vi "Target VI Read.vi"(4 "error in (no error)":errorcluster, 6 "Container State":T2, 7 "Display State In":T1) -> (0 "error out":errorcluster, 2 "Value":path, 3 "Display State Out":T1)   [LabVIEW 2009, in "Jump Button (Modern).xctl"]
uses:
  <vilib>/Navigation Controls/Jump Button/Jump Button (Modern).xctl
  <vilib>/_xctls/Container State.ctl
  <vilib>/Navigation Controls/Jump Button/Jump Button State.ctl
  <vilib>/Navigation Controls/NI_Navigation.lvlib
  <vilib>/_xctls/XControlSupport.lvlib
panel:
  # "Replace the Value Indicator below with an Indicator of desired type.\nDo not remove this Indicator or the others from the connector pane. \nDo not change the connector pane pattern.\nThe Value Indicator should always be the second terminal from top on the output side in the connector pane."
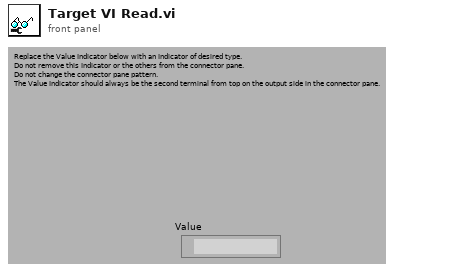
[diagram p1: front panel]
types:
  T1 = typedef "Jump Button (Modern).xctl/Jump Button State.ctl" = cluster{"Button Text":string, "Absolute Path":path, "Relative Path":path}
  T2 = typedef "XControlSupport.lvlib/Container State.ctl" = cluster{"Indicator?":bool, "Run Mode?":bool, " Refnum":refnum<vi>}
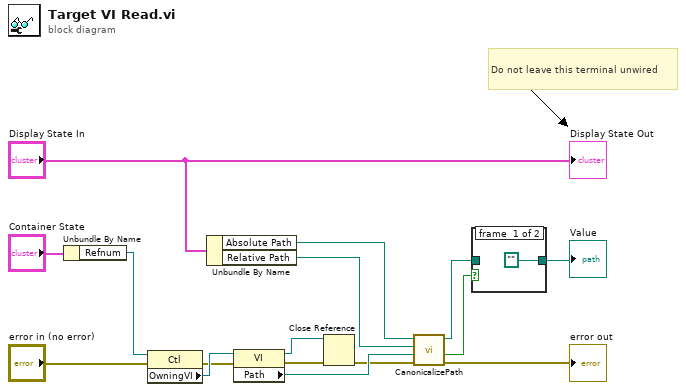
[diagram p0: block diagram]
diagram:
  # "Do not leave this terminal unwired"
  n1 = Unbundle By Name("Container State") -> ("Refnum"=w14:refnum<vi>)
  n2 = property class="Ctl"(reference=w14, error in="error in (no error)") -> (error out=w12:errorcluster, "OwningVI"=w13:refnum<vi>)  [unwired: 1 out]
  n3 = Unbundle By Name("Display State In") -> ("Absolute Path"=w10:path, "Relative Path"=w9:path)
  n4 = property class="VI"(reference=w13, error in=w12) -> (reference out=w4:refnum<vi>, error out=w11:errorcluster, "Path"=w8:path)
  n5 = Close Reference(reference=w4, error in (no error)=w11) -> (error out=w7:errorcluster)
  n6 = call <vilib>:"CanonicalizePath.vi"("error in (no error)"=w7, "VI Path"=w8, "Relative Path"=w9, "Absolute Path"=w10) -> ("error out"=→"error out":errorcluster, "Found?"=w3:bool, "Canonicalized Path Out"=w2:path)  [unwired: 5 in]
  n7 = case shown="False" w3 {
    tunnel: w2 -> [_ w18]
    tunnel: [path "" w18] -> w1
    frame #0 {
    }
    frame #1 {
    }
  }
  "Value" <- w1
  "Display State Out" <- "Display State In"
